vi "FileCanOpen.vi"(6 "提示语":refnum<vi>, 7 "Language":u32, 8 "进度条":refnum<vi>, 9 "进度数值":refnum<vi>, 10 "报文行数统计":refnum<vi>, 11 "file path (dialog if empty)":path caption="文件路径 （空时为对话框）") -> (0 "路径输出":path, 1 "重构的Data数组":u32[][](array[numeric]), 2 "统计数量":string[](array[string]), 3 "报文ID":string[](array[string]), 4 "基时间簇":T1 {"基时间秒" format="%#.6f"}, 5 "CAN报文统计":string[][](array[string]))   [LabVIEW 2015]
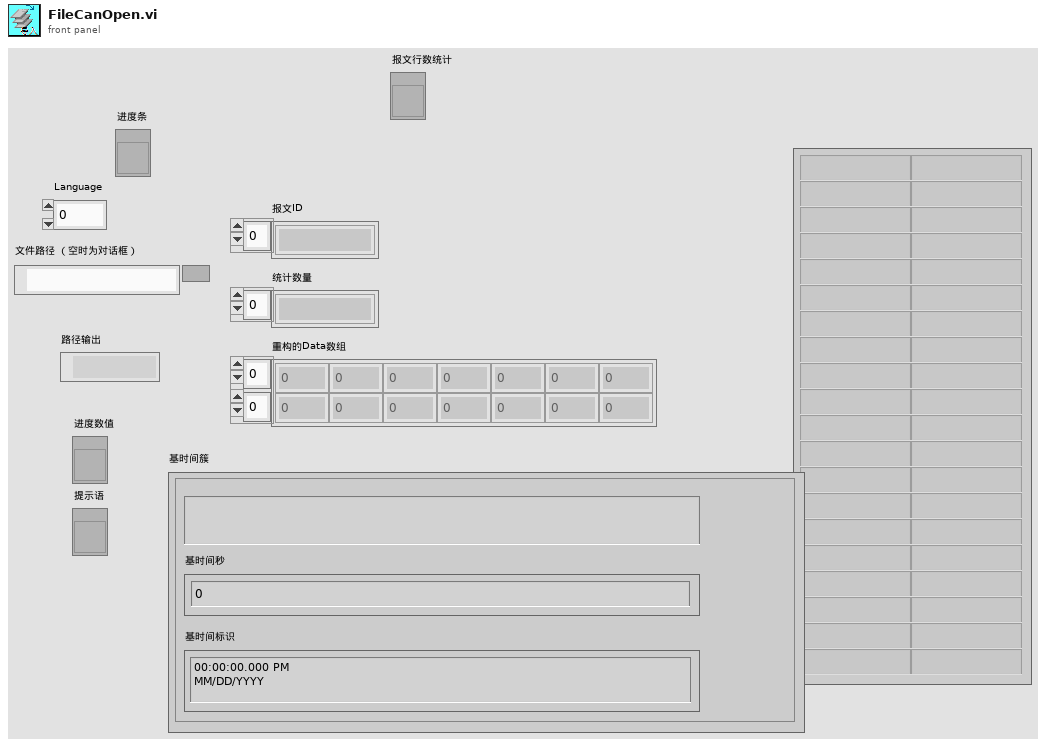
[diagram p1: front panel]
types:
  T1 = cluster{"基时间字符串":string, "基时间秒":dbl, "基时间标识":timestamp}
  T2 = enum16{"open", "replace", "create", "open or create", "replace or create", "replace or create with confirmation"}
  T3 = enum16{"big-endian, network order", "native, host order", "little-endian"}
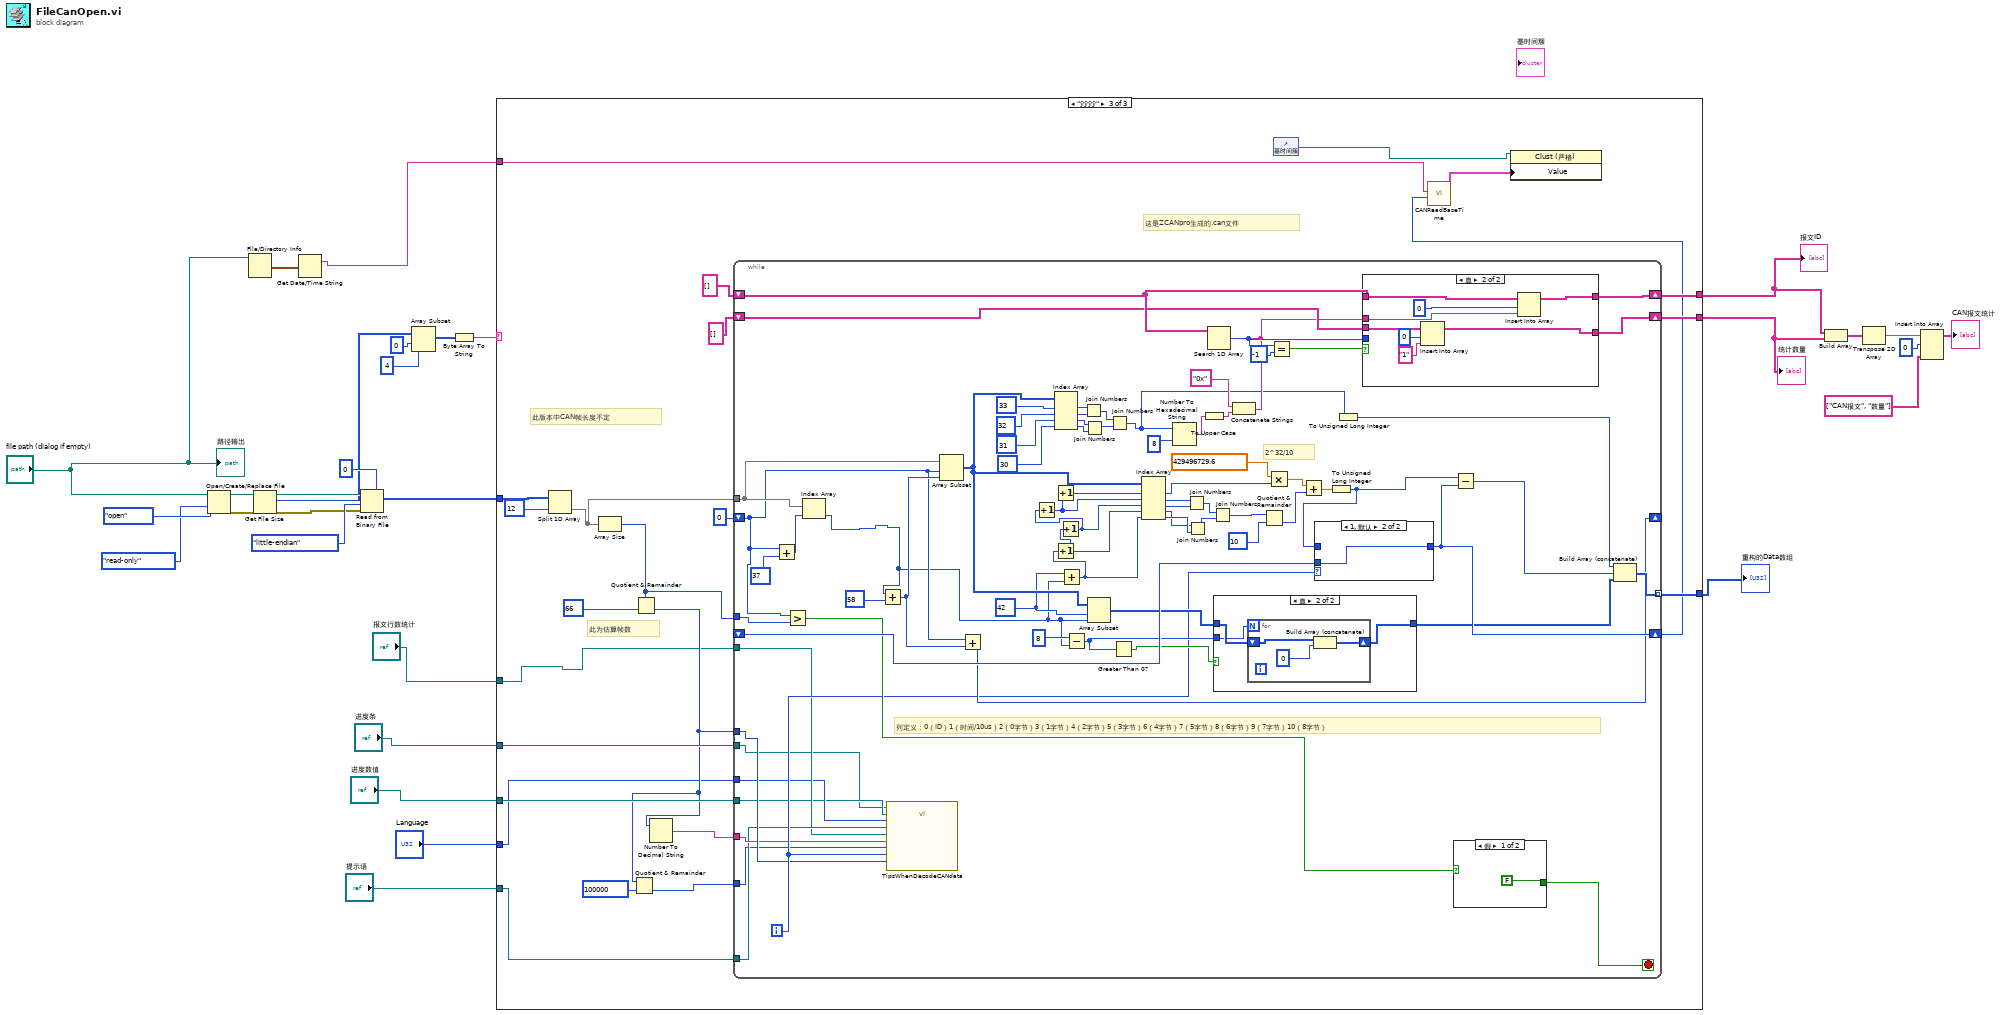
[diagram p0: block diagram]
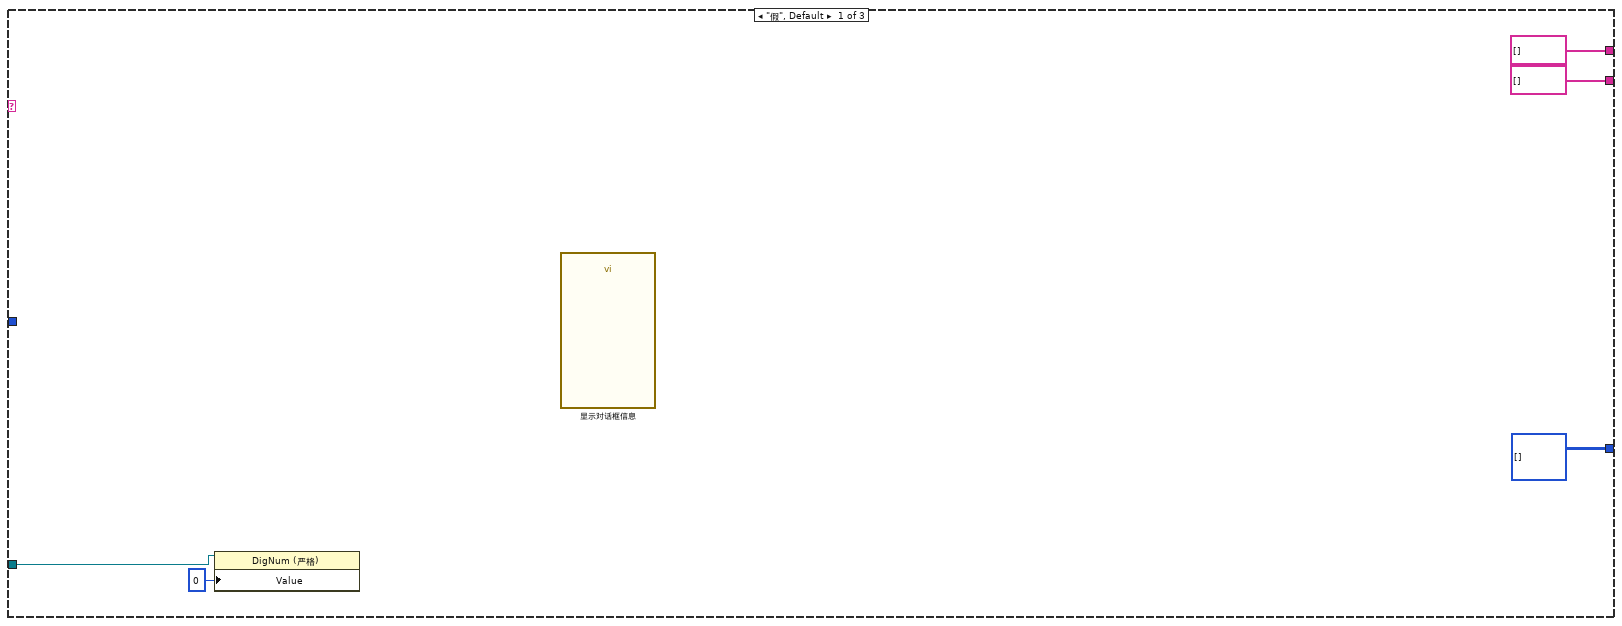
[diagram p2: hidden frame]
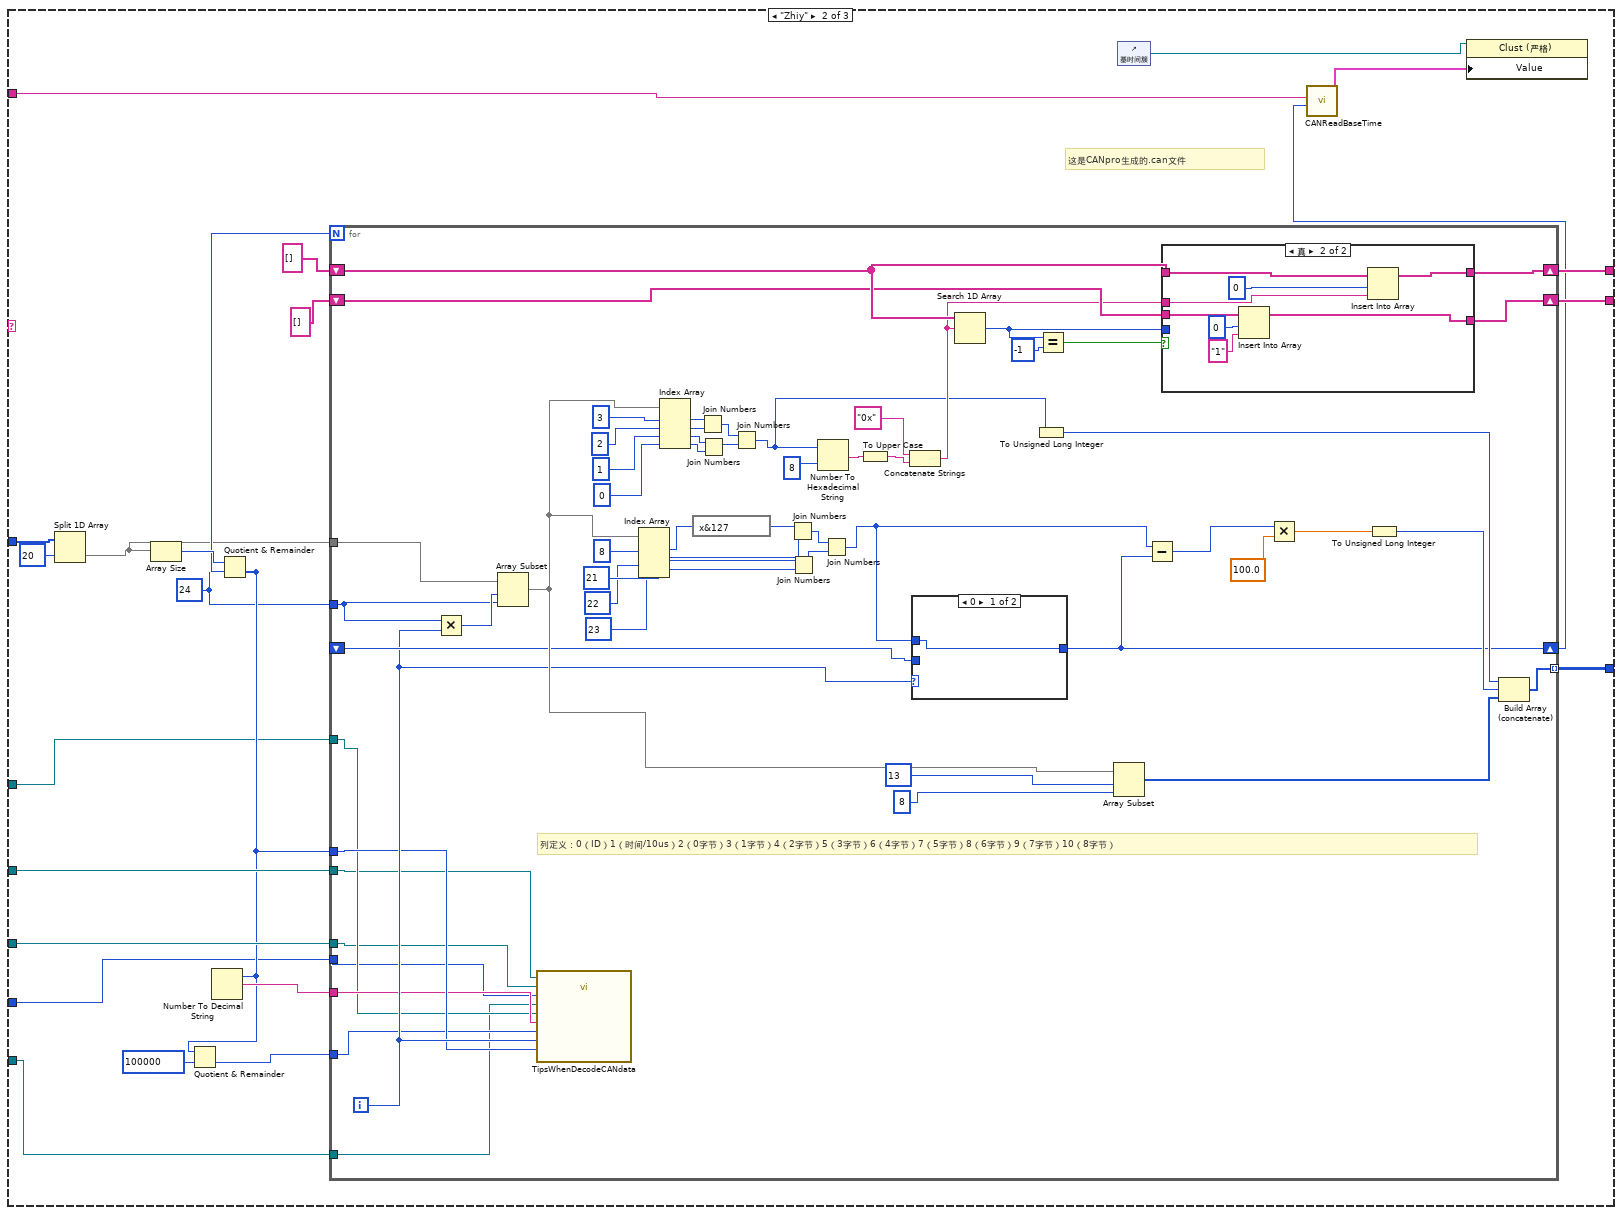
[diagram p3: hidden frame]
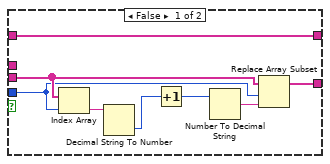
[diagram p5: hidden frame]
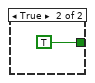
[diagram p6: hidden frame]
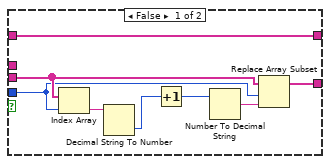
[diagram p9: hidden frame]
diagram:
  n1 = Open/Create/Replace File(file path (use dialog)="file path (dialog if empty)", operation (0:open)=T2."open" ("操作(0:open)"), access (0:read/write)=enum16{"read/write", "read-only", "write-only"}."read-only" ("权限(0:read/write)")) -> (refnum out=w10:refnum<file>, error out=w15:errorcluster)  [unwired: 3 in, 1 out]
  n2 = File/Directory Info(path="file path (dialog if empty)") -> (last mod=w4:timestamp)  [unwired: 1 in, 6 out]
  n3 = Get File Size(file=w10, error in=w15) -> (refnum out=w13:refnum<file>, size (in bytes)=w14:i64, 0:w12:errorcluster)
  n4 = Get Date/Time String(seconds (now)=w4) -> (date string=w2:string)  [unwired: 2 in, 1 out]
  n5 = Read from Binary File(5:u8 0, 8:w12, 9:T3."little-endian" ("字节顺序(0:big-endian, network order)"), 10:w14, 11:w13) -> (2:w6:u8[])  [unwired: 1 in, 3 out]
  n6 = Array Subset(array=w6, index=0 ("索引"), length=4 ("长度")) -> (w7:u8[])
  n7 = Byte Array To String(unsigned byte array=w7) -> (string=w5:string)
  n8 = case shown="\"ÿÿÿÿ\"" w5 {
    tunnel: [u32[][] [] w58 w159] -> w30
    tunnel: [string[] [] w55 w156] -> w25
    tunnel: [string[] [] w54 w155] -> w24
    tunnel: "进度条" -> [_ w53 w154]
    tunnel: "进度数值" -> [_ w52 w153]
    tunnel: "提示语" -> [_ w49 w150]
    tunnel: "报文行数统计" -> [w32 w37 w137]
    tunnel: w6 -> [_ w42 w145]
    tunnel: w2 -> [_ w41 w139]
    tunnel: "Language" -> [_ w36 w136]
    frame "假", Default {
      n9 = property class="DigNum (严格)"(reference=w32, "Value"=0 ("值")) -> ()  [unwired: 1 in, 2 out]
      n10 = call "显示对话框信息"() -> ()  [unwired: 10 in, 2 out]
    }
    frame "Zhiy" {
      w43 = 24 ("y")
      # "这是CANpro生成的.can文件"
      n11 = Split 1D Array(array=w42, index=20 ("索引")) -> (second subarray=w44:u8[])  [unwired: 1 out]
      n12 = Array Size(array=w44) -> (size(s)=w46:i32)
      n13 = Quotient & Remainder(x=w46, y=w43) -> (floor(x/y)=w45:i32)  [unwired: 1 out]
      n14 = Quotient & Remainder(x=w45, y=100000) -> (floor(x/y)=w50:i32)  [unwired: 1 out]
      n15 = Number To Decimal String(number=w45) -> (decimal integer string=w48:string)  [unwired: 1 in]
      n16 = for {
        N: w45 -> [_]
        tunnel: [w117] -> w58 mode=indexing
        shift-right: [w112] -> w55
        shift-left: string[] [] -> [w113]
        shift-right: [w108] -> w54
        shift-left: string[] [] -> [w109]
        tunnel: w45 -> [w66]
        tunnel: w53 -> [w59]
        tunnel: w52 -> [w60]
        tunnel: w50 -> [w65]
        tunnel: w49 -> [w62]
        tunnel: w48 -> [w64]
        tunnel: w44 -> [w105]
        tunnel: w43 -> [w104]
        shift-right: [w73] -> w38
        shift-left: _ -> [w75]
        tunnel: w37 -> [w63]
        tunnel: w36 -> [w61]
        i -> [w67]
        # "列定义：0（ID）1（时间/10us）2（0字节）3（1字节）4（2字节）5（3字节）6（4字节）7（5字节）8（6字节）9（7字节）10（8字节）"
        n17 = Multiply(x=w104, y=w67) -> (x*y=w106:i32)
        n18 = Array Subset(array=w105, index=w106, length=w104) -> (w77:u8[])
        n19 = call "TipsWhenDecodeCANdata.vi"("ProgressBar"=w59, "AllRowsNum"=w66, "i"=w67, "ProgressNum"=w60, "Language"=w61, "Tips"=w62, "MessageLinCnt"=w63, "txtAllRowsNum"=w64, "RowsLevel"=w65) -> ()  [unwired: 7 in]
        n20 = Index Array(array=w77, index #1=8 ("索引"), index #2=21 ("索引"), index #3=22 ("索引"), index #4=23 ("索引")) -> (element #1=w70:u8, element #2=w82:u8, element #3=w81:u8, element #4=w80:u8)
        n21 = Index Array(array=w77, index #1=3 ("索引"), index #2=2 ("索引"), index #3=1 ("索引"), index #4=0 ("索引")) -> (element #1=w99:u8, element #2=w98:u8, element #3=w97:u8, element #4=w96:u8)
        n22 = expression code="x&127"(w70) -> (w69:u8)
        n23 = Join Numbers(hi=w99, lo=w98) -> ((hi.lo)=w95:u16)
        n24 = Join Numbers(hi=w97, lo=w96) -> ((hi.lo)=w94:u16)
        n25 = Join Numbers(hi=w95, lo=w94) -> ((hi.lo)=w90:u32)
        n26 = Join Numbers(hi=w69, lo=w82) -> ((hi.lo)=w83:u16)
        n27 = Join Numbers(hi=w81, lo=w80) -> ((hi.lo)=w84:u16)
        n28 = Number To Hexadecimal String(1:i16 8 ("宽度(-)"), 2:w90) -> (0:w72:string)
        n29 = Join Numbers(hi=w83, lo=w84) -> ((hi.lo)=w74:u32)
        n30 = To Upper Case(1:w72) -> (0:w71:string)
        n31 = Concatenate Strings("0x" ("字符串"), w71) -> (w91:string)
        n32 = case shown="0" w67 {
          tunnel: w74 -> [w118 _]
          tunnel: [w118 w119] -> w73
          tunnel: w75 -> [_ w119]
          frame 0 {
          }
          frame 1, Default {
          }
        }
        n33 = Search 1D Array(1D array=w113, element=w91) -> (index of element=w107:i32)  [unwired: 1 in]
        n34 = To Unsigned Long Integer(number=w90) -> (unsigned 32bit integer=w89:u32)
        n35 = Equal?(x=w107, y=-1) -> (x = y?=w110:bool)
        n36 = Array Subset(array=w77, index=13 ("索引"), length=8 ("索引")) -> (w76:u8[])
        n37 = Subtract(x=w74, y=w73) -> (x-y=w68:u32)
        n38 = case shown="真" w110 {
          tunnel: w113 -> [w127 w135]
          tunnel: [w127 w134] -> w112
          tunnel: w91 -> [_ w133]
          tunnel: w109 -> [w126 w130]
          tunnel: [w125 w131] -> w108
          tunnel: w107 -> [w120 _]
          frame False {
            n39 = Index Array(array=w126, index=w120) -> (element=w124:string)
            n40 = Decimal String To Number(string=w124) -> (number=w123:i32)  [unwired: 2 in, 1 out]
            n41 = Increment(x=w123) -> (x+1=w121:i32)
            n42 = Number To Decimal String(number=w121) -> (decimal integer string=w122:string)  [unwired: 1 in]
            n43 = Replace Array Subset(array=w126, new element=w122, index=w120) -> (w125:string[])
          }
          frame True {
            n44 = Insert Into Array(array=w130, index=0 ("索引"), new element="1" ("新元素/子数组")) -> (w131:string[])
            n45 = Insert Into Array(array=w135, index=0 ("索引"), new element=w133) -> (w134:string[])
          }
        }
        n46 = Multiply(x=w68, y=100.0) -> (x*y=w115:dbl)
        n47 = To Unsigned Long Integer(number=w115) -> (unsigned 32bit integer=w114:u32)
        n48 = Build Array (concatenate)(w89, w114, w76) -> (w117:u32[])
      }
      n49 = control-ref of="基时间簇"() -> (w40:refnum<vi>)
      n50 = call "CANReadBaseTime.vi"("时间"=w38, "日期字符"=w41) -> ("基时间簇"=w39:T1)  [unwired: 7 in]
      n51 = property class="Clust (严格)"(reference=w40, "Value"=w39) -> ()  [unwired: 1 in, 2 out]
    }
    frame "ÿÿÿÿ" {
      # "此为估算帧数"
      # "此版本中CAN帧长度不定"
      # "这是ZCANpro生成的.can文件"
      n52 = Split 1D Array(array=w145, index=12 ("索引")) -> (second subarray=w147:u8[])  [unwired: 1 out]
      n53 = Array Size(array=w147) -> (size(s)=w143:i32)
      n54 = Quotient & Remainder(x=w143, y=66) -> (floor(x/y)=w148:i32)  [unwired: 1 out]
      n55 = Quotient & Remainder(x=w148, y=100000) -> (floor(x/y)=w151:i32)  [unwired: 1 out]
      n56 = Number To Decimal String(number=w148) -> (decimal integer string=w149:string)  [unwired: 1 in]
      n57 = while {
        tunnel: [w233] -> w159 mode=indexing
        shift-right: [w231] -> w156
        shift-left: string[] [] -> [w232]
        shift-right: [w227] -> w155
        shift-left: string[] [] -> [w228]
        tunnel: w148 -> [w167]
        tunnel: w154 -> [w160]
        tunnel: w153 -> [w161]
        tunnel: w151 -> [w164]
        tunnel: w150 -> [w165]
        tunnel: w149 -> [w166]
        tunnel: w147 -> [w191]
        shift-right: [w202] -> w138
        shift-left: _ -> [w203]
        shift-right: [w192] -> _
        shift-left: 0 -> [w186]
        tunnel: w143 -> [w185]
        tunnel: w137 -> [w163]
        tunnel: w136 -> [w162]
        i -> [w168]
        stop <- w172 stop-if-true
        w184 = 42 ("索引")
        # "2^32/10"
        # "列定义：0（ID）1（时间/10us）2（0字节）3（1字节）4（2字节）5（3字节）6（4字节）7（5字节）8（6字节）9（7字节）10（8字节）"
        n58 = Add(x=w186, y=37) -> (x+y=w190:i32)
        n59 = Greater?(x=w186, y=w185) -> (0:w173:bool)
        n60 = Index Array(array=w191, index=w190) -> (element=w171:u8)
        n61 = Add(x=w171, y=u8 58) -> (x+y=w187:u8)
        n62 = call "TipsWhenDecodeCANdata.vi"("ProgressBar"=w160, "AllRowsNum"=w167, "i"=w168, "ProgressNum"=w161, "Language"=w162, "Tips"=w165, "MessageLinCnt"=w163, "txtAllRowsNum"=w166, "RowsLevel"=w164) -> ()  [unwired: 7 in]
        n63 = Array Subset(array=w191, index=w186, length=w187) -> (w204:u8[])
        n64 = Add(x=w186, y=w187) -> (x+y=w192:i32)
        n65 = Index Array(array=w204, index #1=33 ("索引"), index #2=32 ("索引"), index #3=31 ("索引"), index #4=30 ("索引")) -> (element #1=w221:u8, element #2=w220:u8, element #3=w219:u8, element #4=w218:u8)
        n66 = Add(x=w184, y=w171) -> (x+y=w183:i32)
        n67 = Increment(x=w183) -> (x+1=w182:i32)
        n68 = Increment(x=w182) -> (x+1=w181:i32)
        n69 = Increment(x=w181) -> (x+1=w179:i32)
        n70 = Increment(x=w179) -> (x+1=w180:i32)
        n71 = Subtract(x=u8 8 ("y"), y=w171) -> (x-y=w174:u8)
        n72 = Join Numbers(hi=w221, lo=w220) -> ((hi.lo)=w217:u16)
        n73 = Join Numbers(hi=w219, lo=w218) -> ((hi.lo)=w216:u16)
        n74 = Array Subset(array=w204, index=w184, length=w171) -> (w178:u8[])
        n75 = Join Numbers(hi=w217, lo=w216) -> ((hi.lo)=w212:u32)
        n76 = Greater Than 0?(x=w174) -> (x > 0?=w175:bool)
        n77 = Index Array(array=w204, index #1=w180, index #2=w179, index #3=w181, index #4=w182, index #5=w183) -> (element #1=w199:u8, element #2=w205:u8, element #3=w206:u8, element #4=w207:u8, element #5=w208:u8)
        n78 = Number To Hexadecimal String(1:i16 8 ("宽度(-)"), 2:w212) -> (0:w170:string)
        n79 = Join Numbers(hi=w205, lo=w206) -> ((hi.lo)=w209:u16)
        n80 = Join Numbers(hi=w207, lo=w208) -> ((hi.lo)=w210:u16)
        n81 = To Upper Case(1:w170) -> (0:w169:string)
        n82 = Join Numbers(hi=w209, lo=w210) -> ((hi.lo)=w201:u32)
        n83 = case shown="真" w175 {
          tunnel: w178 -> [w236 w239]
          tunnel: [w236 w238] -> w177
          tunnel: w174 -> [_ w237]
          frame False {
          }
          frame True {
            n84 = for {
              N: w237 -> [_]
              shift-right: [w241] -> w238
              shift-left: w239 -> [w240]
              n85 = Build Array (concatenate)(w240, u8 0) -> (w241:u8[])
            }
          }
        }
        n86 = Concatenate Strings("0x" ("字符串"), w169) -> (w213:string)
        n87 = Search 1D Array(1D array=w232, element=w213) -> (index of element=w226:i32)  [unwired: 1 in]
        n88 = Quotient & Remainder(x=w201, y=u32 10) -> (floor(x/y)=w196:u32)  [unwired: 1 out]
        n89 = Multiply(x=429496729.6, y=w199) -> (x*y=w197:dbl)
        n90 = Equal?(x=w226, y=-1) -> (x = y?=w229:bool)
        n91 = Add(x=w197, y=w196) -> (x+y=w195:dbl)
        n92 = To Unsigned Long Integer(number=w195) -> (unsigned 32bit integer=w194:u32)
        n93 = case shown="1, 默认" w168 {
          tunnel: w194 -> [w243 _]
          tunnel: [w243 w244] -> w202
          tunnel: w203 -> [_ w244]
          frame 0 {
          }
          frame 1, Default {
          }
        }
        n94 = To Unsigned Long Integer(number=w212) -> (unsigned 32bit integer=w211:u32)
        n95 = case shown="真" w229 {
          tunnel: w232 -> [w252 w260]
          tunnel: [w252 w259] -> w231
          tunnel: w213 -> [_ w258]
          tunnel: w228 -> [w251 w255]
          tunnel: [w250 w256] -> w227
          tunnel: w226 -> [w245 _]
          frame False {
            n96 = Index Array(array=w251, index=w245) -> (element=w249:string)
            n97 = Decimal String To Number(string=w249) -> (number=w248:i32)  [unwired: 2 in, 1 out]
            n98 = Increment(x=w248) -> (x+1=w246:i32)
            n99 = Number To Decimal String(number=w246) -> (decimal integer string=w247:string)  [unwired: 1 in]
            n100 = Replace Array Subset(array=w251, new element=w247, index=w245) -> (w250:string[])
          }
          frame True {
            n101 = Insert Into Array(array=w255, index=0 ("索引"), new element="1" ("新元素/子数组")) -> (w256:string[])
            n102 = Insert Into Array(array=w260, index=0 ("索引"), new element=w258) -> (w259:string[])
          }
        }
        n103 = case shown="假" w173 {
          tunnel: [FALSE TRUE] -> w172
          frame False {
          }
          frame True {
          }
        }
        n104 = Subtract(x=w194, y=w202) -> (x-y=w193:u32)
        n105 = Build Array (concatenate)(w211, w193, w177) -> (w233:u32[])
      }
      n106 = control-ref of="基时间簇"() -> (w140:refnum<vi>)
      n107 = call "CANReadBaseTime.vi"("时间"=w138, "日期字符"=w139) -> ("基时间簇"=w141:T1)  [unwired: 7 in]
      n108 = property class="Clust (严格)"(reference=w140, "Value"=w141) -> ()  [unwired: 1 in, 2 out]
    }
  }
  "重构的Data数组" <- w30
  "报文ID" <- w25
  "统计数量" <- w24
  n109 = Build Array(w25, w24) -> (w29:string[][])
  n110 = Transpose 2D Array(2D array=w29) -> (transposed array=w28:string[][])
  n111 = Insert Into Array(array=w28, index (row)=0 ("索引 (行)"), new element=string[] ["CAN报文", "数量"]) -> (→"CAN报文统计":string[][])  [unwired: 1 in]
  "路径输出" <- "file path (dialog if empty)"
